vi "Example IMAQdx Cam and XDisplay Step 3.vi"() -> ()   [LabVIEW 2014]
uses:
  <vilib>/userdefined/High Color/IMAQdx.ctl
  XDisplay/POLARIS IMAQ Display.xctl
  IMAQdx Cam/IMAQdx Cam.lvclass
  Analyze Classes/Analyze Fluence/Analyze Fluence.lvclass
  Analyze Classes/Analyze Q-Factor/Analyze q-Factor.lvclass
  Analyze Classes/Analyze Distanz/Analyze Distanz.lvclass
panel:
  in  "WorkDir":path
  in  "ConfigDir":path
  in  "XDisplay":cluster{"Image":T1}(xcontrol)
  in  "Show Settings":bool
  in  "File Prefix":string
  in  "Energy":dbl[unit]
  in  "Camera":T2="JustageCam"
  in  "stop":bool
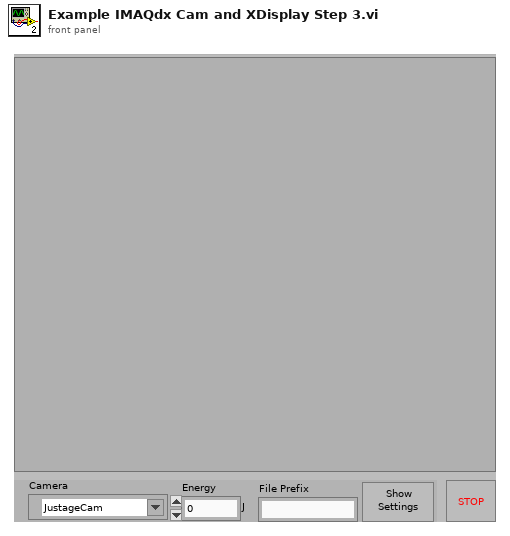
[diagram p1: front panel]
types:
  T1 = typedef "IMAQ Image.ctl" = refnum<image>
  T2 = typedef "IMAQdx.ctl" = refnum<k21>
  T3 = cluster{"Desired Font (Application)":enum16{"User-specified Font", "Application Font", "System Font", "Dialog Font"}, "[User-specified Font]":cluster{"Font Name":string, "Size":i16, "Strikeout?":bool, "Italic?":bool, "Underline?":bool, "Outline?":bool, "Shadow?":bool, "Bold?":bool, "Rotation Angle":dbl}, "Horizontal Alignment":i16, "Vertical Alignment":i16}
  T4 = typedef "Image Type" = u32
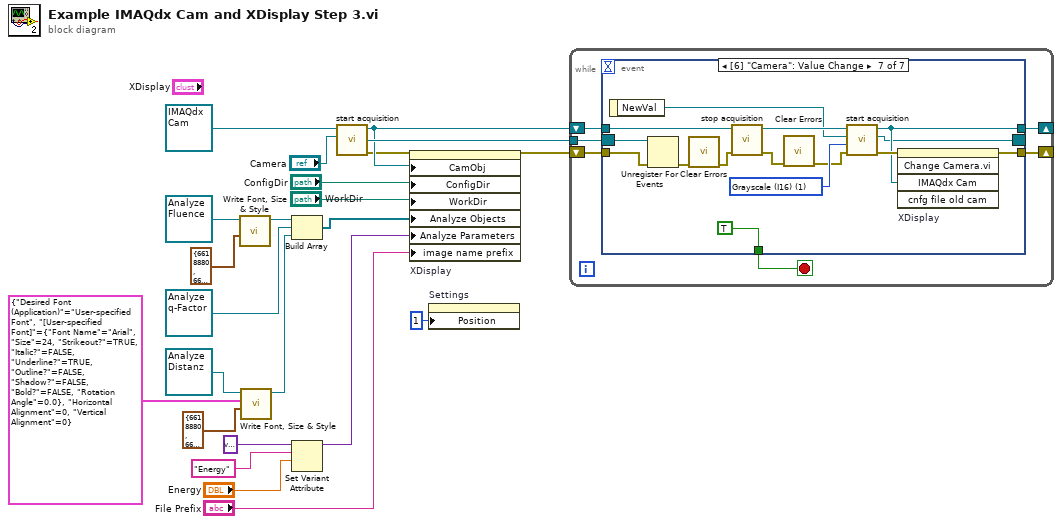
[diagram p0: block diagram]
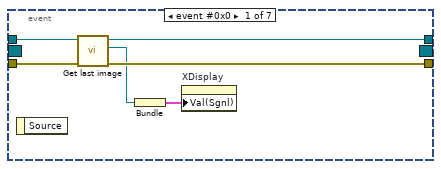
[diagram p2: hidden frame]
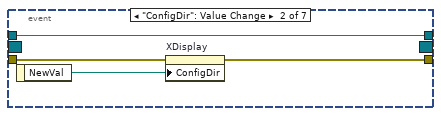
[diagram p3: hidden frame]
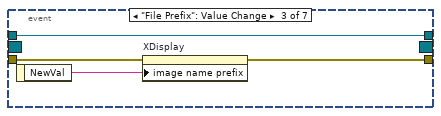
[diagram p4: hidden frame]
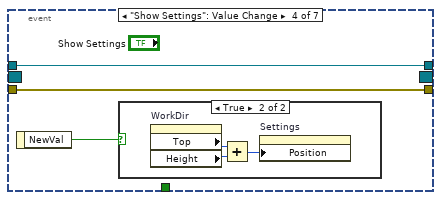
[diagram p5: hidden frame]
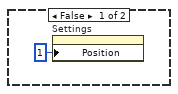
[diagram p6: hidden frame]
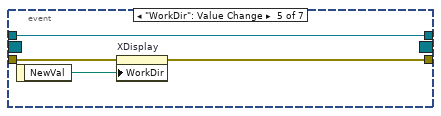
[diagram p7: hidden frame]
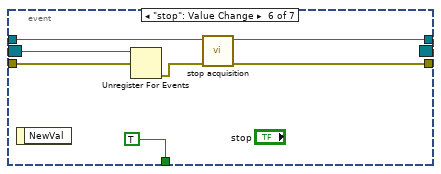
[diagram p8: hidden frame]
diagram:
  n1 = call-dynamic "Write Font, Size & Style.vi"("Overlay colors"=cluster{"Border":u32, "Text":u32} {"Border"=6618880, "Text"=6618880}, "Analyze BaseClass in"=refnum<class "Analyze Fluence.lvclass"> refnum ("Analyze.lvlib:Analyze Fluence.lvclass")) -> ("Analyze BaseClass out"=w8:refnum<class "Analyze Fluence.lvclass">)  [unwired: 8 in, 1 out]
  n2 = call-dynamic "Write Font, Size & Style.vi"("Overlay colors"=cluster{"Border":u32, "Text":u32} {"Border"=6618880, "Text"=6618880}, "Font, Size & Style"=T3 {"Desired Font (Application)"=enum."User-specified Font", "[User-specified Font]"={"Font Name"="Arial", "Size"=24, "Strikeout?"=TRUE, "Italic?"=FALSE, "Underline?"=TRUE, "Outline?"=FALSE, "Shadow?"=FALSE, "Bold?"=FALSE, "Rotation Angle"=0.0}, "Horizontal Alignment"=0, "Vertical Alignment"=0}, "Analyze BaseClass in"=refnum<class "Analyze Distanz.lvclass"> refnum ("Analyze.lvlib:Analyze Distanz.lvclass")) -> ("Analyze BaseClass out"=w5:refnum<class "Analyze Distanz.lvclass">)  [unwired: 7 in, 1 out]
  n3 = Build Array(w8, refnum<class "Analyze q-Factor.lvclass"> refnum ("Analyze.lvlib:Analyze q-Factor.lvclass"), w5) -> (w14:refnum<class "Analyze BaseClass.lvclass">[])
  n4 = Set Variant Attribute(Variant=variant ("Analyze Parameters"), name="Energy", value="Energy") -> (Variant out=w12:variant)  [unwired: 1 in, 2 out]
  n5 = call-dynamic "start acquisition.vi"("Camera Name"="Camera", "IMAQdx Cam in"=refnum<class "IMAQdx Cam.lvclass"> refnum ("IMAQdx Cam.lvclass")) -> ("error out"=w19:errorcluster, "Event Registration Refnum"=w22:refnum<event-registration>, "IMAQdx Cam out"=w20:refnum<class "IMAQdx Cam.lvclass">)  [unwired: 7 in]
  n6 = property on="XDisplay" class="POLARIS IMAQ Display (strict)"(error in=w19, "CamObj"=w20, "ConfigDir"="ConfigDir", "WorkDir"="WorkDir", "Analyze Objects"=w14, "Analyze Parameters"=w12, "image name prefix"="File Prefix") -> (error out=w18:errorcluster)  [unwired: 1 in, 1 out]
  n7 = property on="Settings" class="Splitter"("Position"=1 ("Splitter Position")) -> ()  [unwired: 2 in, 2 out]
  n8 = while {
    tunnel: w22 -> [w24]
    shift-right: [w27] -> _
    shift-left: w20 -> [w29]
    shift-right: [w26] -> _
    shift-left: w18 -> [w28]
    stop <- w25 stop-if-true
    n9 = event shown="[6] \"Camera\": Value Change" {
      selector: w24 -> [_ _ _ _ _ w60 w75]
      dyn-events: [_ _ _ _ _ _ w63] -> _
      timeout: _ -> [_ _ _ _ _ _ _]
      tunnel: w29 -> [w35 w39 w43 w45 w54 w58 w73]
      tunnel: w28 -> [w34 w37 w41 w44 w52 w59 w74]
      tunnel: [w33 w39 w43 w45 w54 w56 w64] -> w27
      tunnel: [w32 w36 w40 w44 w51 w55 w62] -> w26
      tunnel: [_ _ _ _ _ TRUE TRUE] -> w25
      event event #0x0 {
        n10 = event-data() -> ()  [unwired: 1 in, 1 out]
        n11 = call-dynamic "Get last image.vi"("error in (no error)"=w34, "IMAQdx Cam in"=w35) -> ("error out"=w32:errorcluster, "Image Out"=w31:T1, "IMAQdx Cam out"=w33:refnum<class "IMAQdx Cam.lvclass">)  [unwired: 6 in, 1 out]
        n12 = Bundle("Image Out"=w31) -> (w30:cluster{"Image Out":T1})  [unwired: 1 in]
        n13 = property on="XDisplay" class="POLARIS IMAQ Display (strict)"("Val(Sgnl)"=w30) -> ()  [unwired: 2 in, 2 out]
      }
      event "ConfigDir": Value Change {
        n14 = event-data() -> ("NewVal"=w38:path)  [unwired: 1 in]
        n15 = property on="XDisplay" class="POLARIS IMAQ Display (strict)"(error in=w37, "ConfigDir"=w38) -> (error out=w36:errorcluster)  [unwired: 1 in, 1 out]
      }
      event "File Prefix": Value Change {
        n16 = event-data() -> ("NewVal"=w42:string)  [unwired: 1 in]
        n17 = property on="XDisplay" class="POLARIS IMAQ Display (strict)"(error in=w41, "image name prefix"=w42) -> (error out=w40:errorcluster)  [unwired: 1 in, 1 out]
      }
      event "Show Settings": Value Change {
        n18 = event-data() -> ("NewVal"=w46:bool)  [unwired: 1 in]
        n19 = case shown="True" w46 {
          frame False {
            n20 = property on="Settings" class="Splitter"("Position"=1 ("Splitter Position")) -> ()  [unwired: 2 in, 2 out]
          }
          frame True {
            n21 = property on="WorkDir" class="Path"() -> ("Top"=w50:i32, "Height"=w49:u32)  [unwired: 2 in, 2 out]
            n22 = Add(x=w50, y=w49) -> (x+y=w48:u32)
            n23 = property on="Settings" class="Splitter"("Position"=w48) -> ()  [unwired: 2 in, 2 out]
          }
        }
      }
      event "WorkDir": Value Change {
        n24 = event-data() -> ("NewVal"=w53:path)  [unwired: 1 in]
        n25 = property on="XDisplay" class="POLARIS IMAQ Display (strict)"(error in=w52, "WorkDir"=w53) -> (error out=w51:errorcluster)  [unwired: 1 in, 1 out]
      }
      event "stop": Value Change {
        n26 = event-data() -> ()  [unwired: 1 in, 1 out]
        n27 = Unregister For Events(event registration refnum=w60, error in=w59) -> (error out=w57:errorcluster)
        n28 = call-dynamic "stop acquisition.vi"("error in (no error)"=w57, "IMAQdx Cam in"=w58) -> ("error out"=w55:errorcluster, "IMAQdx Cam out"=w56:refnum<class "IMAQdx Cam.lvclass">)  [unwired: 8 in]
      }
      event Value Change {
        w72 = T4 1 items=["Grayscale (U8)", "Grayscale (I16)", "Grayscale (SGL)", "Complex (CSG)", "RGB (U32)", "HSL (U32)", "RGB (U64)", "Grayscale (U16)"] ("Image Type")
        n29 = event-data() -> ("NewVal"=w66:T2)  [unwired: 1 in]
        n30 = Unregister For Events(event registration refnum=w75, error in=w74) -> (error out=w69:errorcluster)
        n31 = call <vilib>:"Clear Errors.vi"("error in (no error)"=w69) -> ("error out"=w68:errorcluster)  [unwired: 5 in, 1 out]
        n32 = call-dynamic "stop acquisition.vi"("error in (no error)"=w68, "IMAQdx Cam in"=w73) -> ("error out"=w70:errorcluster, "IMAQdx Cam out"=w67:refnum<class "IMAQdx Cam.lvclass">)  [unwired: 8 in]
        n33 = call <vilib>:"Clear Errors.vi"("error in (no error)"=w70) -> ("error out"=w71:errorcluster)  [unwired: 5 in, 1 out]
        n34 = call-dynamic "start acquisition.vi"("error in (no error)"=w71, "Image Type"=w72, "Camera Name"=w66, "IMAQdx Cam in"=w67) -> ("error out"=w65:errorcluster, "Event Registration Refnum"=w63:refnum<event-registration>, "IMAQdx Cam out"=w64:refnum<class "IMAQdx Cam.lvclass">)  [unwired: 5 in]
        n35 = invoke on="XDisplay" class="POLARIS IMAQ Display (strict)" method="Change Camera.vi"(error in=w65, "IMAQdx Cam"=w64) -> (error out=w62:errorcluster)  [unwired: 3 in, 4 out]
      }
    }
  }
